vi "init.vi"(8 "error in (no error)":errorcluster, 11 "IRQHandler in":refnum<class "IRQHandler.lvclass">) -> (0 "error out":errorcluster, 3 "IRQHandler out":refnum<class "IRQHandler.lvclass">)   [LabVIEW 2013, in "ComponentData.lvlib" / "IRQHandler.lvclass"]
uses:
  <userlib>/Common/Component/common_application/RT/ComponentData/IRQHandler/IRQHandler.lvclass
  <userlib>/Common/Component/common_application/RT/ComponentData/IRQHandler/IRQHandler.lvclass/IRQHandler.ctl
  <userlib>/Common/Component/common_application/RT/ComponentData/ConfigurationHandler/IRQConfig/IRQConfig.lvclass
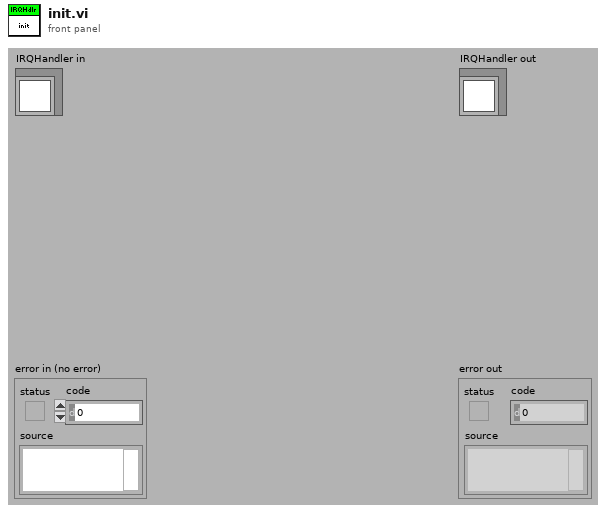
[diagram p1: front panel]
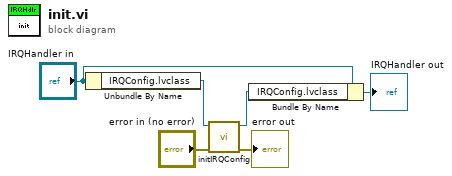
[diagram p0: block diagram]
diagram:
  n1 = Unbundle By Name("IRQHandler in") -> ("IRQConfig.lvclass"=w2:refnum<class "IRQConfig.lvclass">)
  n2 = call <userlib>:"initIRQConfig.vi"("error in (no error)"="error in (no error)", "IRQConfig in"=w2) -> ("error out"=→"error out":errorcluster, "IRQConfig out"=w1:refnum<class "IRQConfig.lvclass">)  [unwired: 8 in]
  n3 = Bundle By Name(cluster="IRQHandler in", "IRQConfig.lvclass"=w1) -> (→"IRQHandler out":refnum<class "IRQHandler.lvclass">)
